vi "Create Server SMO.vi"(6 "Debug Mode?":bool, 8 "error in (no error)":errorcluster, 9 "Commands":string[](array[string]), 10 "Port":u16, 11 "RemoteControl in":refnum<class "RemoteControl.lvclass">) -> (0 "error out":errorcluster, 3 "RemoteControl out":refnum<class "RemoteControl.lvclass">)   [LabVIEW 2019, in "RemoteControl.lvlib" / "RemoteControl.lvclass"]
uses:
  RemoteControl.lvclass
  <vilib>/JKI/JKI SMO/SMO/SMO.lvclass
  Typedefs/RC Process Type--Enum.ctl
  <vilib>/JKI/JKI SMO/SMO/Typedefs/SMOState --Enum.ctl
  <vilib>/JKI/JKI SMO/SMO/Typedefs/Public Events.ctl
  Typedefs/Message--Cluster.ctl
  Typedefs/PublicEvents--RemoteControl.SendMessageFromProcess.ctl
  Typedefs/PublicEvents--Cluster.ctl
  <userlib>/LevyLab/Debug/Debug.lvlib
  <userlib>/LevyLab/Debug/Attribute.Debug/DebugBehavior.ctl
  <userlib>/LevyLab/Debug/Attribute.Debug/Attribute.Debug.lvclass
  <vilib>/JKI/JKI SMO/SMO/Typedefs/Reserve State--Enum.ctl
  C:/Program Files (x86)/National Instruments/LabVIEW 2019/vi.lib/JKI/JKI SMO/SMO/SMO.lvclass
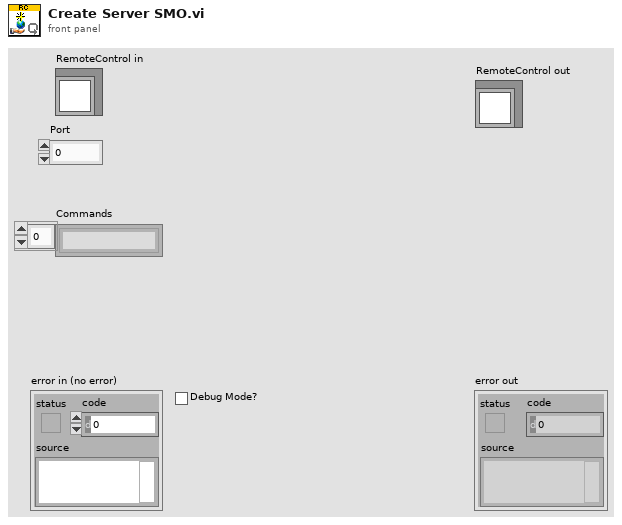
[diagram p1: front panel]
types:
  T1 = typedef "Debug.lvlib/Attribute.Debug.lvclass/DebugBehavior.ctl" = enum16{"Normal", "Debug"}
  T2 = typedef "RemoteControl.lvlib/RemoteControl.lvclass/RC Process Type--Enum.ctl" = enum16{"Listener", "Server", "Client"}
  T3 = typedef "RemoteControl.lvlib/RemoteControl.lvclass/PublicEvents--Cluster.ctl" = cluster{"SendMessageFromProcess":refnum<user-event>}
  T4 = typedef "smo.lvlib/SMO.lvclass/Public Events.ctl" = cluster{"Error":refnum<user-event>, "State":refnum<user-event>, "Reserve State":refnum<user-event>}
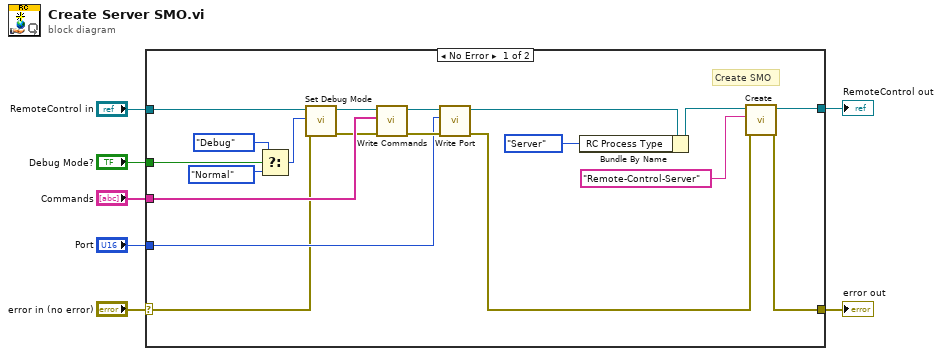
[diagram p0: block diagram]
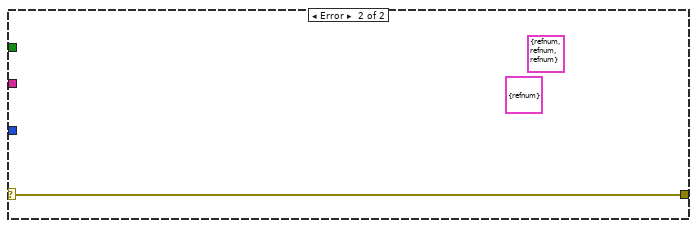
[diagram p2: hidden frame]
diagram:
  n1 = case shown="No Error" "error in (no error)" {
    selector: "error in (no error)" -> [w10 w27]
    tunnel: [w25 w27] -> w6
    tunnel: [w26 _] -> w5
    tunnel: "Commands" -> [w18 _]
    tunnel: "Port" -> [w17 _]
    tunnel: "RemoteControl in" -> [w9 _]
    tunnel: "Debug Mode?" -> [w11 _]
    frame No Error {
      # "Create SMO"
      n2 = Select(t=DebugBehavior."Debug" ("Behavior"), s=w11, f=DebugBehavior."Normal" ("Behavior")) -> (s? t:f=w12:T1)
      n3 = call <userlib>:"Set Debug Mode.vi"("error in (no error)"=w10, "Behavior"=w12, "SMO"=w9) -> ("error out"=w15:errorcluster, "SMO out"=w8:refnum<class "RemoteControl.lvclass">)  [unwired: 7 in]
      n4 = call-dynamic "Write Commands.vi"("error in (no error)"=w15, "Commands"=w18, "RemoteControl in"=w8) -> ("error out"=w21:errorcluster, "RemoteControl out"=w20:refnum<class "RemoteControl.lvclass">)  [unwired: 7 in]
      n5 = call-dynamic "Write Port.vi"("error in (no error)"=w21, "Port"=w17, "RemoteControl in"=w20) -> ("error out"=w19:errorcluster, "RemoteControl out"=w16:refnum<class "RemoteControl.lvclass">)  [unwired: 7 in]
      n6 = Bundle By Name(cluster=w16, "RC Process Type"=RC_Process_Type--Enum."Server") -> (w23:refnum<class "RemoteControl.lvclass">)
      n7 = call <vilib>:"Create.vi"("error in (no error)"=w19, "Subsystem Name (optional)"="Remote-Control-Server" ("format string"), "SMO"=w23) -> ("error out"=w25:errorcluster, "SMO out"=w26:refnum<class "RemoteControl.lvclass">)  [unwired: 6 in, 1 out]
    }
    frame Error {
      (unwired) T3 {"SendMessageFromProcess"=refnum} ("RC Public Events")
      (unwired) T4 {"Error"=refnum, "State"=refnum, "Reserve State"=refnum} ("Public Events")
    }
  }
  "error out" <- w6
  "RemoteControl out" <- w5
